vi "Create Project Item - VI.vi"(8 "Error In":errorcluster, 11 "ProjectItem Refnum":refnum<vi>) -> (0 "Error Passthrough":errorcluster, 1 "Error During VI Project Item Creation":errorcluster, 2 "Project Item Out":T1, 3 "ProjectItem Refnum Out":refnum<vi>)   [LabVIEW 2014, in "i3-docs.lvlib"]
uses:
  i3-docs.lvlib
  Controls/project_item.ctl
  Controls/image_information.ctl
  Controls/config_fgv_actions.ctl
  <vilib>/Utility/error.llb/Error Cluster From Error Code.vi
  <vilib>/ErrorRing/Error Ring.xnode
  <vilib>/Utility/NIReport.llb/NI_ReportGenerationCore.lvlib
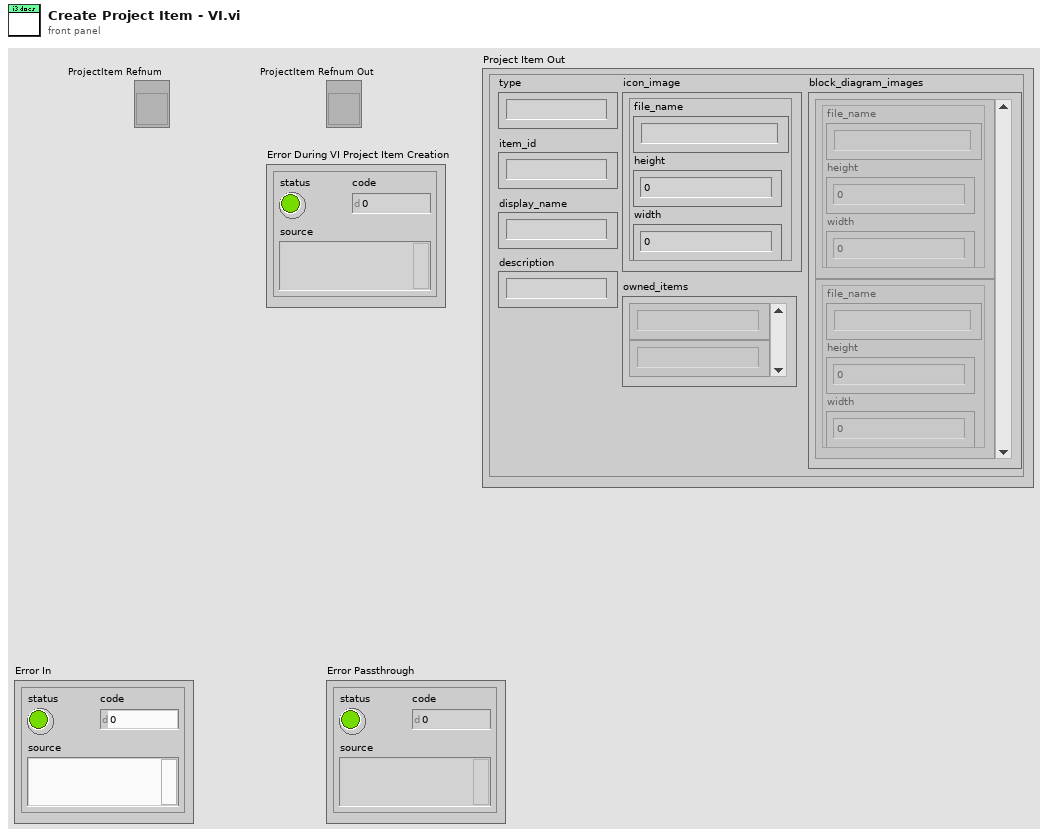
[diagram p1: front panel]
types:
  T1 = typedef "i3-docs.lvlib/project_item.ctl" = cluster{"type":string, "owned_items":string[], "item_id":string, "display_name":string, "description":string, "block_diagram_images":T2[], "icon_image":T2}
  T2 = typedef "i3-docs.lvlib/image_information.ctl" = cluster{"file_name":string, "height":i32, "width":i32}
  T3 = typedef "i3-docs.lvlib/config_fgv_actions.ctl" = enum16{"Initialize", "Set Current Project", "Get Current Config", "Set Current Project Item", "Finished"}
  T4 = cluster{"Printing:Custom All Controls?":bool, "Printing:Custom Connector?":bool, "Printing:Custom Control Descriptions?":bool, "Printing:Custom Control Types?":bool, "Printing:Custom Controls?":bool, "Printing:Custom Description?":bool, "Printing:Custom Diagram Hidden?":bool, "Printing:Custom Diagram Repeat?":bool, "Printing:Custom Diagram?":bool, "Printing:Custom Hierarchy?":bool, "Printing:Custom History?":bool, "Printing:Custom Panel Border?":bool, "Printing:Custom Panel?":bool, "Printing:Custom SubVIs?":bool}
  T5 = typedef "i3-docs.lvlib/current_config.ctl" = cluster{"project file":path, "output directory":path}
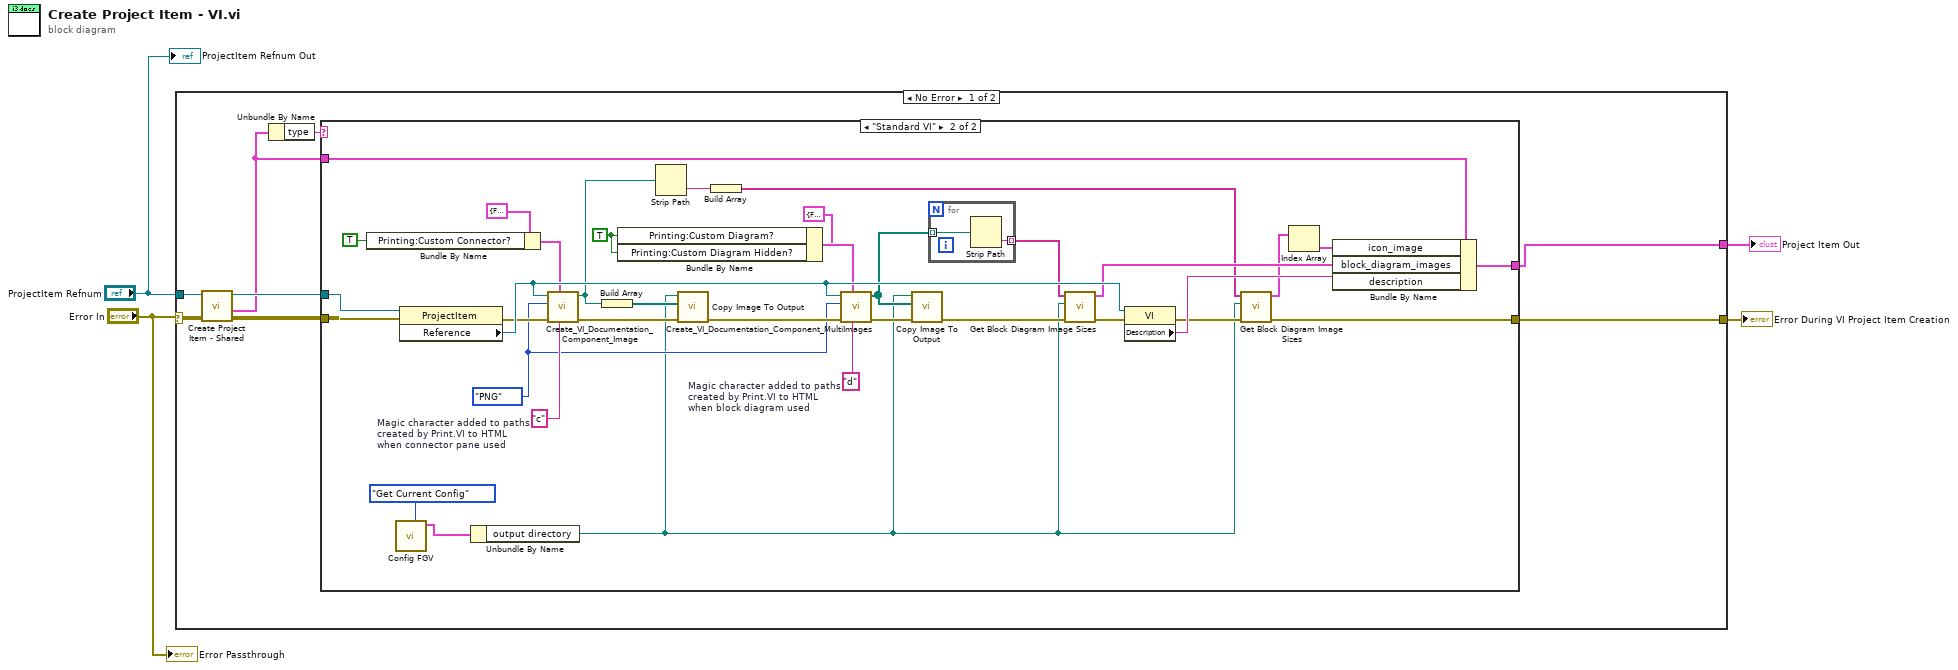
[diagram p0: block diagram]
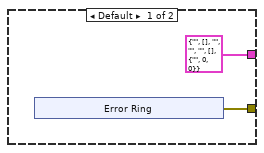
[diagram p2: hidden frame]
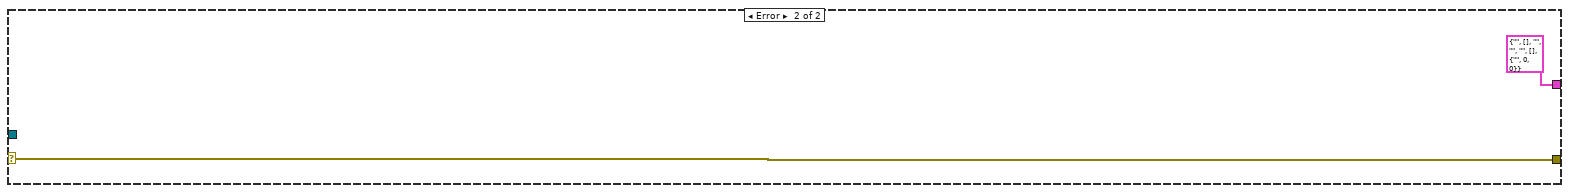
[diagram p3: hidden frame]
diagram:
  n1 = case shown="No Error" "Error In" {
    selector: "Error In" -> [w9 w58]
    tunnel: [w12 w58] -> w4
    tunnel: "ProjectItem Refnum" -> [w8 _]
    tunnel: [w11 T1 {"type"="", "owned_items"=[], "item_id"="", "display_name"="", "description"="", "block_diagram_images"=[], "icon_image"={"file_name"="", "height"=0, "width"=0}} ("project_item")] -> w2
    frame No Error {
      n2 = call "Create Project Item - Shared.vi"("Error In"=w9, "ProjectItem Refnum"=w8) -> ("Error Out"=w10:errorcluster, "project_item"=w5:T1, "ProjectItem Refnum Out"=w6:refnum<vi>)  [unwired: 6 in, 1 out]
      n3 = Unbundle By Name(w5) -> ("type"=w7:string)
      n4 = case shown="\"Standard VI\"" w7 {
        tunnel: w10 -> [_ w52]
        tunnel: w6 -> [_ w51]
        tunnel: [w14 w25] -> w12
        tunnel: [T1 {"type"="", "owned_items"=[], "item_id"="", "display_name"="", "description"="", "block_diagram_images"=[], "icon_image"={"file_name"="", "height"=0, "width"=0}} ("project_item") w49] -> w11
        tunnel: w5 -> [_ w50]
        frame Default {
          n5 = xnode "Error Ring"() -> ("error out"=w14:errorcluster)
        }
        frame "Standard VI" {
          w35 = TRUE ("Printing:Custom Diagram?")
          w40 = "d"  # Magic character added to paths created by Print.VI to HTML when block diagram used
          w42 = enum32{"PNG", "JPEG", "GIF"}."PNG" ("Image Format (jpeg)")
          w47 = "c"  # Magic character added to paths created by Print.VI to HTML when connector pane used
          n6 = Bundle By Name(cluster=T4 {"Printing:Custom All Controls?"=FALSE, "Printing:Custom Connector?"=FALSE, "Printing:Custom Control Descriptions?"=FALSE, "Printing:Custom Control Types?"=FALSE, "Printing:Custom Controls?"=FALSE, "Printing:Custom Description?"=FALSE, "Printing:Custom Diagram Hidden?"=FALSE, "Printing:Custom Diagram Repeat?"=FALSE, "Printing:Custom Diagram?"=FALSE, "Printing:Custom Hierarchy?"=FALSE, "Printing:Custom History?"=FALSE, "Printing:Custom Panel Border?"=FALSE, "Printing:Custom Panel?"=FALSE, "Printing:Custom SubVIs?"=FALSE} ("Content Options"), "Printing:Custom Connector?"=TRUE) -> (w45:T4)
          n7 = call "Config FGV.vi"("Action"=config_fgv_actions."Get Current Config") -> ("Current Project Configuration"=w32:T5)  [unwired: 8 in, 2 out]
          n8 = property class="ProjectItem"(reference=w51, error in=w52) -> (error out=w48:errorcluster, "Reference"=w54:refnum<vi>)  [unwired: 1 out]
          n9 = Unbundle By Name(w32) -> ("output directory"=w24:path)
          n10 = call <vilib>:"Create_VI_Documentation_Component_Image.vi"("special chars in file path of image"=w47, "Content Options"=w45, "error in (no error)"=w48, "Image Format (jpeg)"=w42, "VI"=w54) -> ("error out"=w44:errorcluster, "Path to image"=w36:path)  [unwired: 5 in]
          n11 = Build Array(w36) -> (w34:path[])
          n12 = Bundle By Name(cluster=T4 {"Printing:Custom All Controls?"=FALSE, "Printing:Custom Connector?"=FALSE, "Printing:Custom Control Descriptions?"=FALSE, "Printing:Custom Control Types?"=FALSE, "Printing:Custom Controls?"=FALSE, "Printing:Custom Description?"=FALSE, "Printing:Custom Diagram Hidden?"=FALSE, "Printing:Custom Diagram Repeat?"=FALSE, "Printing:Custom Diagram?"=FALSE, "Printing:Custom Hierarchy?"=FALSE, "Printing:Custom History?"=FALSE, "Printing:Custom Panel Border?"=FALSE, "Printing:Custom Panel?"=FALSE, "Printing:Custom SubVIs?"=FALSE} ("Content Options"), "Printing:Custom Diagram?"=w35, "Printing:Custom Diagram Hidden?"=w35) -> (w39:T4)
          n13 = Strip Path(path=w36) -> (name=w23:string)  [unwired: 1 out]
          n14 = call "Copy Image To Output.vi"("Error In"=w44, "Paths to copy"=w34, "Directory to copy to"=w24) -> ("Error Out"=w43:errorcluster)  [unwired: 8 in]
          n15 = Build Array(w23) -> (w22:string[])
          n16 = call <vilib>:"Create_VI_Documentation_Component_MultiImages.vi"("special chars in file path of image"=w40, "Content Options"=w39, "error in (no error)"=w43, "Image Format (jpeg)"=w42, "VI"=w54) -> ("error out"=w41:errorcluster, "Paths to images"=w33:path[])  [unwired: 5 in]
          n17 = call "Copy Image To Output.vi"("Error In"=w41, "Paths to copy"=w33, "Directory to copy to"=w24) -> ("Error Out"=w30:errorcluster)  [unwired: 8 in]
          n18 = for {
            tunnel: w33 -> [w56] mode=indexing
            tunnel: [w55] -> w28 mode=indexing
            n19 = Strip Path(path=w56) -> (name=w55:string)  [unwired: 1 out]
          }
          n20 = call "Get Block Diagram Image Sizes.vi"("Error In"=w30, "Images Directory"=w24, "Image Names"=w28) -> ("Error Out"=w29:errorcluster, "Block Diagram Images"=w27:T2[])  [unwired: 7 in]
          n21 = property class="VI"(reference=w54, error in=w29) -> (error out=w26:errorcluster, "Description"=w53:string)  [unwired: 1 out]
          n22 = call "Get Block Diagram Image Sizes.vi"("Error In"=w26, "Images Directory"=w24, "Image Names"=w22) -> ("Error Out"=w25:errorcluster, "Block Diagram Images"=w21:T2[])  [unwired: 7 in]
          n23 = Index Array(array=w21) -> (element=w20:T2)  [unwired: 1 in]
          n24 = Bundle By Name(cluster=w50, "icon_image"=w20, "block_diagram_images"=w27, "description"=w53) -> (w49:T1)
        }
      }
    }
    frame Error {
    }
  }
  "Error During VI Project Item Creation" <- w4
  "Project Item Out" <- w2
  "ProjectItem Refnum Out" <- "ProjectItem Refnum"
  "Error Passthrough" <- "Error In"
